vi "Monitor_setBoolean.vi"(0 "ColorModule":cluster{u32, u32}[](array[cluster]), 1 "ControlName":string, 2 "Tab Control":refnum<vi>, 3 "Boolean in":refnum<vi>) -> ()   [LabVIEW 2015]
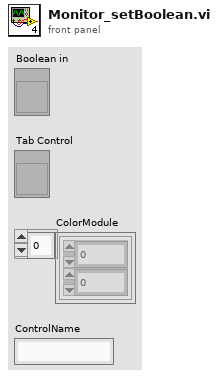
[diagram p1: front panel]
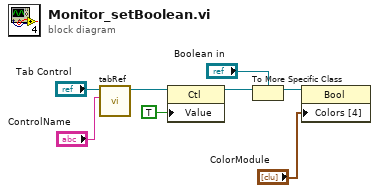
[diagram p0: block diagram]
diagram:
  n1 = call "tabRef.vi"("control name"="ControlName", "Tab Control"="Tab Control") -> ("control refnum"=w1:refnum<vi>)  [unwired: 8 in, 1 out]
  n2 = property class="Ctl"(reference=w1, "Value"=TRUE) -> (reference out=w6:refnum<vi>)  [unwired: 1 in, 1 out]
  n3 = To More Specific Class(target class="Boolean in", reference=w6) -> (specific class reference=w7:refnum<vi>)  [unwired: 1 in, 1 out]
  n4 = property class="Bool"(reference=w7, "Colors [4]"="ColorModule") -> ()  [unwired: 1 in, 2 out]
